vi "USRP Dummy DMA Fetch Whatever (Host).vi"() -> ()   [LabVIEW 2016]
uses:
  <vilib>/userdefined/High Color/nirio_resource_hc.ctl
  <vilib>/FPGAPlugInAG/USRP 294xR; 295xR 200 MSps/niLvFpga_Open_USRP 294xR; 295xR 200 MSps.vi
  <vilib>/rvi/interface/common/dynamic/niFpgaDynamicAddResources.vi
  <vilib>/FPGAPlugInAG/Dynamic/niLvFpga_Download_Dynamic.vi
  <vilib>/FPGAPlugInAG/Dynamic/niLvFpga_Run_Dynamic.vi
  <vilib>/Utility/error.llb/Error Cluster From Error Code.vi
  <vilib>/rvi/errors/niLvFpgaAdjustHostInterfaceError.vi
  <vilib>/rvi/interface/common/niFpgaWaitOnOcc.vi
  <vilib>/FPGAPlugInAG/Dynamic/niLvFpga_Close_Dynamic.vi
  <vilib>/rvi/interface/nirviOpenFPGA/nirviOpenFPGA.xnode
  FPGA Bitfiles/USRP-RIO-Streami_DummyDMA_USRPDummyv2(FPGA_kYza4iCu9yA.lvbitx
  <vilib>/rvi/interface/nirviMethod/nirviMethod.xnode
  <vilib>/rvi/interface/nirviReadWriteControl/nirviReadWriteControl.xnode
  <vilib>/rvi/interface/nirviCloseFPGA/nirviCloseFPGA.xnode
  <vilib>/rvi/errors/niLvFpgaMergeErrorWithErrorCode.vi
  <vilib>/rvi/interface/Simulation/niFpgaSimulationCallBeginRW.vi
  <instrlib>/niUsrpRio/Config/v1/Host/niUsrpRio Config v1 Host.lvlib
  NiFpgaLv.dll
  <vilib>/FPGAPlugInAG/Dynamic/niLvFpga_StopFifo_Dynamic.vi
  <vilib>/FPGAPlugInAG/Dynamic/niLvFpga_ConfigureFifo_Dynamic.vi
  <vilib>/FPGAPlugInAG/Dynamic/niLvFpga_StartFifo_Dynamic.vi
  <vilib>/FPGAPlugInAG/Dynamic/niLvFpga_ReadFifo_Dynamic.vi
panel:
  out "Host Transfer Slider":u64(slide) scale=0.0..68719476736.0
  in  "Flush FIFO?":bool
  out "Control Loop":i32
  in  "Host FIFO Max Fetch":u32=131072
  in  "Reset Host Count?":bool
  in  "Stop Transfer?":bool
  in  "Reset FPGA Count?":bool
  out "FPGA Side FIFO":cluster{u32, u32}(slide)={66, 63} scale=0.0..2047.0
  out "Host Side FIFO":cluster{u32, u32}(slide) scale=0.0..67108863.0
  out "Data Loop":i32
  out "Fetch Loop":i32
  out "Host Count":u64
  in  "Number of Samples":u64=68719476736
  out "FPGA Count":u64
  in  "Start Transfer":bool
  in  "stop":bool
  out "Elements Remaining":u32
  out "Data":u64[](array[numeric]) format="%016x"
  out "Timeout Counts":u64
  in  "Reset Timeouts?":bool
  out "Actual Depth":u32
  in  "Host Requested Depth":u32=67108864
  out "error out":errorcluster
  in  "error in (no error)":errorcluster
  in  "resource name":T1="PXI2Slot18Port1Dev1"
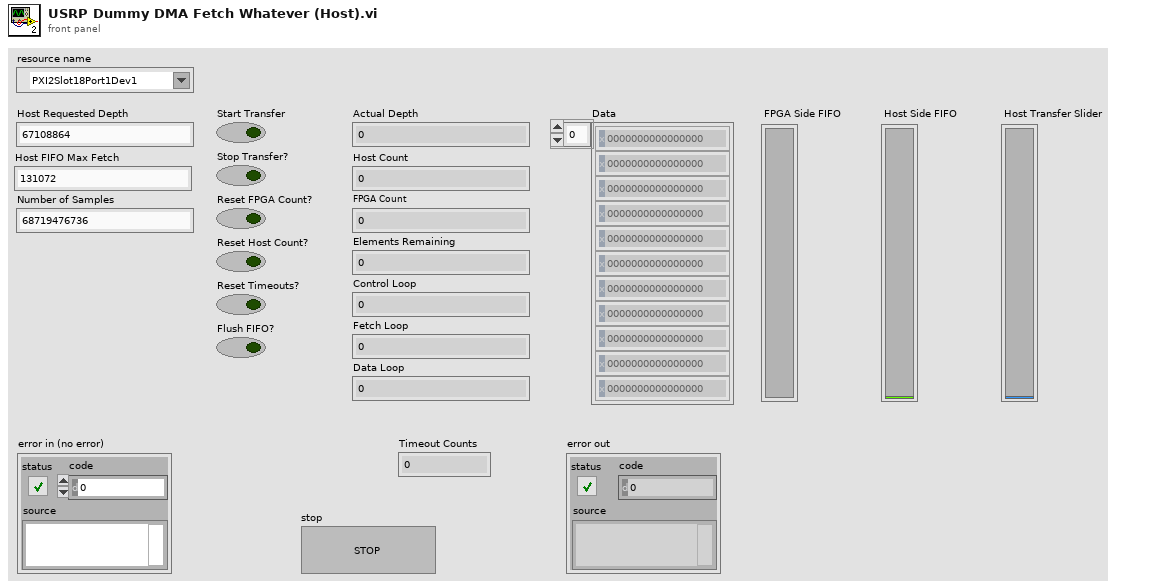
[diagram p1: front panel]
types:
  T1 = typedef "nirio_resource_hc.ctl" = tag
  T2 = typedef "niUsrpRio Config v1 Host.lvlib/niUsrpRio Session.ctl" = cluster{"FPGA Interface":refnum<k20>, "RIO Interface Number":u32, "Data Clock Rate":u32, "FPGA Data Clock Rate":u32, "Global Settings Register Bus":T3, "Radio 0 Settings Register Bus":T3, "Radio 1 Settings Register Bus":T3, "Radio Settings Bus Semaphore":T4, "DB Queues":T5[], "Characterization Data Valid?":bool, "EEPROM Header":T6, "Device Data Header":T7, "EEPROM Characterization Header":T8, "Characterization Data":T9[], "FPGA Current Version":u32, "FPGA Oldest Compatible Version":u32, "Fixed Logic Current Version":u32, "Fixed Logic Oldest Compatible Version":u32, "FPGA Radio Settings Bus Current Version":u32, "FPGA Radio Settings Bus Oldest Compatible Version":u32, "FPGA Board Config Current Version":u32, "FPGA Board Config Oldest Compatible Version":u32, "Daughterboard Clock Rate":u32, "daughterboard configuration session handles":u64[]}
  T3 = typedef "niInstr Register Bus v0 Host.lvlib/Register Bus Session.ctl" = refnum<queue>
  T4 = typedef "Semaphore RefNum" = refnum<k1>
  T5 = typedef "niUsrpRio Config v1 Host.lvlib/DB Queue Reference.ctl" = refnum<queue>
  T6 = typedef "niUsrpRio Config v1 Host.lvlib/EEPROM Header.ctl" = cluster{"Checksum":u32, "Product Code":u16, "Hardware Current Version":u16, "Hardware Oldest Compatible Version":u16, "EEPROM Map Current Version":u16, "EEPROM Map Oldest Compatible Version":u16, "User Password":string, "Pointer to Factory Header":u32, "Pointer to User Header":u32, "Recommended Interval":u16, "Number of Reserved Bytes":i32, "Number of Daughterboards":u8, "Daughterboard IDs":u16[], "Daughterboard Serial Numbers":string[]}
  T7 = typedef "niUsrpRio Config v1 Host.lvlib/EEPROM Device Data Header.ctl" = cluster{"Checksum":u32, "Number of Channels":u8, "Number of Gain Settings":u16[], "Pointer to Characterization Data":u32[], "Number of Reserved Bytes":i32, "Number of Frequencies":u16[]}
  T8 = typedef "niUsrpRio Config v1 Host.lvlib/EEPROM Characterization Header.ctl" = cluster{"Checksum":u32, "Date":timestamp, "Temperature":sgl, "Misc. Info":string, "Pointer to Device Data Header":u32, "Number of Reserved Bytes":i32}
  T9 = typedef "niUsrpRio Config v1 Host.lvlib/Characterization Data.ctl" = cluster{"Gains[dB]":dbl[], "Frequencies [Hz]":dbl[], "IQ Imbalance Table":T10[], "Measured Gains[dB]":dbl[][]}
  T10 = typedef "niUsrpRio Config v1 Host.lvlib/IQ Imbalance.ctl" = cluster{"Gain Imbalance [linear]":dbl, "Phase Imbalance [radians]":dbl, "Offset":cdb}
  T11 = cluster{"Maximum Amount Used":u32, "Current Amount Used":u32}
  T12 = cluster{"Running Max":u32, "Elements Remaining":u32}
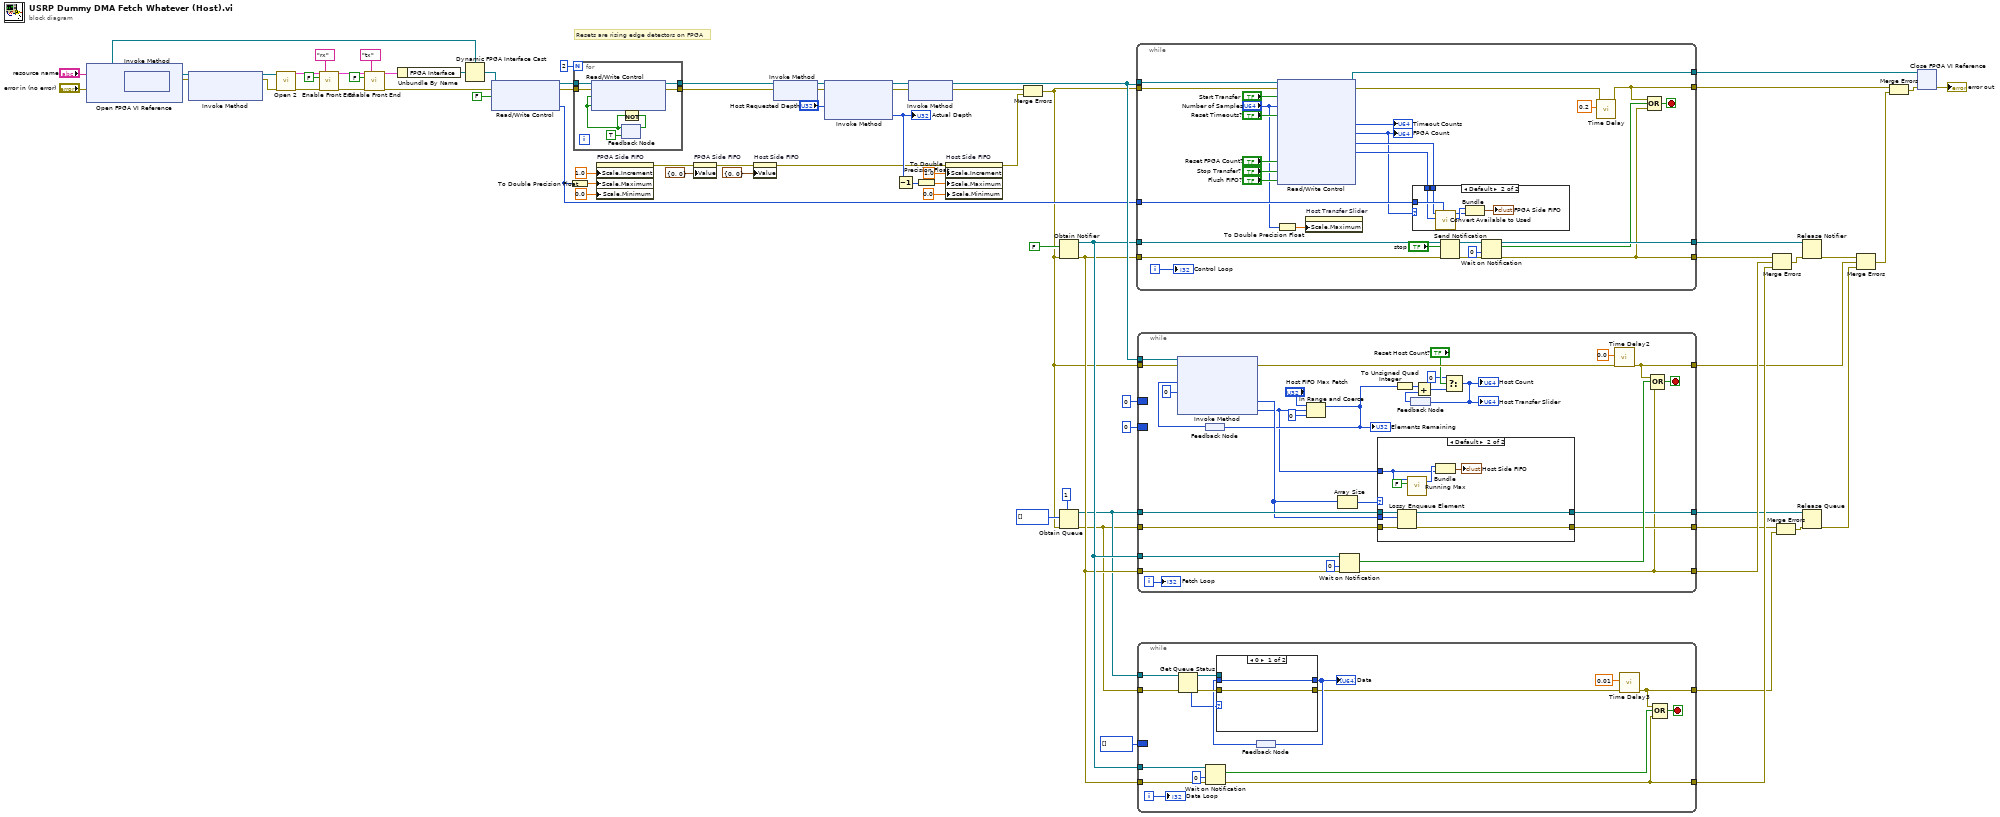
[diagram p0: block diagram]
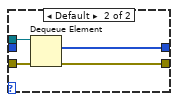
[diagram p2: hidden frame]
diagram:
  # "Resets are rising edge detectors on FPGA"
  n1 = xnode "Open FPGA VI Reference"("error in"="error in (no error)", "resource name"="resource name") -> ("FPGA VI Reference Out"=w6:refnum<k20>, "error out"=w5:errorcluster)
  n2 = xnode "Invoke Method"("FPGA VI Reference In"=w6, "error in"=w5) -> ("FPGA VI Reference Out"=w4:refnum<k20>, "error out"=w3:errorcluster)
  n3 = xnode "Invoke Method"("FPGA VI Reference In"=w4, "error in"=w3) -> ("FPGA VI Reference Out"=w2:refnum<k20>, "error out"=w1:errorcluster)  [unwired: 1 in]
  n4 = call <instrlib>:"Open 2.vi"("fpga ref"=w2, "error in"=w1) -> ("niUsrpRio Session (out)"=w65:T2, "error out"=w70:errorcluster)  [unwired: 12 in]
  n5 = call <instrlib>:"Enable Front End.vi"("niUsrpRio Session"=w65, "scope"="rx", "enable"=FALSE, "error in"=w70) -> ("niUsrpRio Session (out)"=w66:T2, "error out"=w69:errorcluster)  [unwired: 10 in]
  n6 = call <instrlib>:"Enable Front End.vi"("niUsrpRio Session"=w66, "scope"="tx", "enable"=FALSE, "error in"=w69) -> ("niUsrpRio Session (out)"=w62:T2, "error out"=w61:errorcluster)  [unwired: 10 in]
  n7 = Unbundle By Name(w62) -> ("FPGA Interface"=w60:refnum<k20>)
  n8 = Dynamic FPGA Interface Cast(Session In=w6, Type=w60) -> (Session Out=w59:refnum<k20>)
  n9 = xnode "Read/Write Control"("FPGA VI Reference In"=w59, "error in"=w61, "Start Transfer?"=FALSE ("send data?")) -> ("FPGA VI Reference Out"=w35:refnum<k20>, "error out"=w34:errorcluster, "FPGA FIFO Depth"=w20:u32)
  n10 = To Double Precision Float(number=w20) -> (double precision float=w22:dbl)
  n11 = for {
    N: 2 -> [_]
    tunnel: w35 -> [w83]
    tunnel: w34 -> [w82]
    tunnel: [w81] -> w33
    tunnel: [w80] -> w32
    n12 = feedback #1(TRUE) -> (w78:bool)
    n13 = xnode "Read/Write Control"("FPGA VI Reference In"=w83, "error in"=w82, "Reset Timeouts?"=w78, "Reset FPGA Count?"=w78) -> ("FPGA VI Reference Out"=w81:refnum<k20>, "error out"=w80:errorcluster)
    n14 = Not(x=w78) -> (.not. x?=w77:bool)
    n15 = feedback-in #1(w77) -> ()
  }
  n16 = property on="FPGA Side FIFO" class="Slide (strict)"("Scale.Increment"=1.0 ("Scale.Range:Increment"), "Scale.Maximum"=w22, "Scale.Minimum"=0.0 ("Scale.Range:Minimum")) -> (error out=w15:errorcluster)  [unwired: 2 in, 1 out]
  n17 = property on="FPGA Side FIFO" class="Slide (strict)"(error in=w15, "Value"=cluster{u32, u32} {0, 0} ("FPGA Side FIFO")) -> (error out=w18:errorcluster)  [unwired: 1 in, 1 out]
  n18 = property on="Host Side FIFO" class="Slide (strict)"(error in=w18, "Value"=cluster{u32, u32} {0, 0} ("FPGA Side FIFO")) -> (error out=w14:errorcluster)  [unwired: 1 in, 1 out]
  n19 = xnode "Invoke Method"("FPGA VI Reference In"=w33, "error in"=w32) -> ("FPGA VI Reference Out"=w76:refnum<k20>, "error out"=w75:errorcluster)
  n20 = xnode "Invoke Method"("FPGA VI Reference In"=w76, "error in"=w75, "Requested Depth"="Host Requested Depth") -> ("FPGA VI Reference Out"=w72:refnum<k20>, "error out"=w73:errorcluster, "Actual Depth"=w19:u32)
  "Actual Depth" <- w19
  n21 = Decrement(x=w19) -> (x-1=w25:u32)
  n22 = xnode "Invoke Method"("FPGA VI Reference In"=w72, "error in"=w73) -> ("FPGA VI Reference Out"=w56:refnum<k20>, "error out"=w21:errorcluster)
  n23 = To Double Precision Float(number=w25) -> (double precision float=w7:dbl)
  n24 = property on="Host Side FIFO" class="Slide (strict)"(error in=w14, "Scale.Increment"=1.0 ("Data Entry Limits:Increment"), "Scale.Maximum"=w7, "Scale.Minimum"=0.0 ("Data Entry Limits:Minimum")) -> (error out=w12:errorcluster)  [unwired: 1 in, 1 out]
  n25 = Merge Errors(w21, w12) -> (w13:errorcluster)
  n26 = Obtain Notifier(notification data type=FALSE, error in (no error)=w13) -> (notifier out=w47:refnum<notifier>, error out=w46:errorcluster)  [unwired: 2 in, 1 out]
  n27 = Obtain Queue(max queue size (-1, unlimited)=1, element data type=u64[] [] ("Data"), error in (no error)=w13) -> (queue out=w39:refnum<queue>, error out=w38:errorcluster)  [unwired: 2 in, 1 out]
  n28 = while {
    tunnel: w56 -> [w112]
    tunnel: w13 -> [w111]
    tunnel: w47 -> [w108]
    tunnel: w46 -> [w107]
    tunnel: [w102] -> w52
    tunnel: [w95] -> w51
    tunnel: [w97] -> w30
    tunnel: [w96] -> w29
    tunnel: w20 -> [w94]
    i -> [w87]
    stop <- w101 stop-if-true
    n29 = xnode "Read/Write Control"("FPGA VI Reference In"=w112, "error in"=w111, "Start Transfer?"="Start Transfer", "Number of Samples"="Number of Samples", "Reset Timeouts?"="Reset Timeouts?", "Reset FPGA Count?"="Reset FPGA Count?", "Stop Transfer?"="Stop Transfer?", "Flush FIFO?"="Flush FIFO?") -> ("FPGA VI Reference Out"=w96:refnum<k20>, "error out"=w110:errorcluster, "Timeout Count"=→"Timeout Counts":u64, "FPGA Count"=w88:u64, "Space Available"=w93:u32, "Min Space Available"=w91:u32)
    "FPGA Count" <- w88
    n30 = To Double Precision Float(number="Number of Samples") -> (double precision float=w84:dbl)
    n31 = property on="Host Transfer Slider" class="Slide (strict)"("Scale.Maximum"=w84) -> ()  [unwired: 2 in, 2 out]
    n32 = case shown="Default" w88 {
      tunnel: w94 -> [_ w118]
      tunnel: w93 -> [_ w117]
      tunnel: w91 -> [_ w116]
      frame 0 {
      }
      frame Default {
        n33 = call "Convert Available to Used.vi"("Size"=w118, "Minimum Amount Available"=w116, "Current Amount Available"=w117) -> ("Maximum Amount Used"=w115:u32, "Current Amount Used"=w114:u32)  [unwired: 5 in]
        n34 = Bundle("Maximum Amount Used"=w115, "Current Amount Used"=w114) -> (→"FPGA Side FIFO":T11)  [unwired: 1 in]
      }
    }
    n35 = Send Notification(notification="stop", notifier=w108, error in (no error)=w107) -> (notifier out=w104:refnum<notifier>, error out=w103:errorcluster)
    n36 = Wait on Notification(notifier=w104, timeout in ms (-1)=0, error in (no error)=w103) -> (notifier out=w102:refnum<notifier>, notification=w100:bool, error out=w95:errorcluster)  [unwired: 1 in, 1 out]
    n37 = call "Time Delay"("error in (no error)"=w110, "Delay Time (s)"=0.2) -> ("error out"=w97:errorcluster)  [unwired: 9 in]
    n38 = Compound Arithmetic op=OR(w97, w100, w95) -> (w101:bool)
    "Control Loop" <- w87
  }
  n39 = while {
    tunnel: [w143] -> w31
    tunnel: w56 -> [w146]
    tunnel: w13 -> [w145]
    border: u64 0 -> [_]
    border: u32 0 ("Elements Remaining") -> [_]
    tunnel: w47 -> [w139]
    tunnel: w46 -> [w138]
    tunnel: [w128] -> w49
    tunnel: [w134] -> w43
    tunnel: w39 -> [w135]
    tunnel: w38 -> [w133]
    tunnel: [w132] -> w42
    i -> [w136]
    stop <- w141 stop-if-true
    n40 = feedback #2() -> (w124:u32)
    n41 = xnode "Invoke Method"("FPGA VI Reference In"=w146, "error in"=w145, "Number of Elements"=w124, "Timeout (ms)"=0) -> ("error out"=w131:errorcluster, "Data"=w129:u64[], "Elements Remaining"=w119:u32)  [unwired: 1 out]
    n42 = In Range and Coerce(upper limit="Host FIFO Max Fetch", x=w119, lower limit=u32 0) -> (coerced(x)=w121:u32)  [unwired: 1 out]
    "Elements Remaining" <- w121
    n43 = feedback-in #2(w121) -> ()
    n44 = Array Size(array=w129) -> (size(s)=w130:i32)
    n45 = Wait on Notification(notifier=w139, timeout in ms (-1)=0, error in (no error)=w138) -> (notification=w137:bool, error out=w128:errorcluster)  [unwired: 1 in, 2 out]
    n46 = case shown="Default" w130 {
      tunnel: w135 -> [w150 w159]
      tunnel: [w150 w158] -> w134
      tunnel: w133 -> [w149 w157]
      tunnel: [w149 w156] -> w132
      tunnel: w129 -> [_ w155]
      tunnel: w119 -> [_ w151]
      frame 0 {
      }
      frame Default {
        n47 = Lossy Enqueue Element(queue=w159, element=w155, error in (no error)=w157) -> (queue out=w158:refnum<queue>, error out=w156:errorcluster)  [unwired: 2 out]
        n48 = call "Running Max.vi"("Reset"=FALSE, "Next Value"=w151) -> ("Running Max"=w152:u32)  [unwired: 5 in]
        n49 = Bundle("Running Max"=w152, "Elements Remaining"=w151) -> (→"Host Side FIFO":T12)  [unwired: 1 in]
      }
    }
    n50 = To Unsigned Quad Integer(1:w121) -> (0:w148:u64)
    n51 = feedback #3() -> (w147:u64)
    n52 = Add(x=w148, y=w147) -> (x+y=w126:u64)
    n53 = Select(t=u64 0, s="Reset Host Count?", f=w126) -> (s? t:f=w120:u64)
    "Host Count" <- w120
    "Host Transfer Slider" <- w120
    n54 = feedback-in #3(w120) -> ()
    n55 = call "Time Delay2"("error in (no error)"=w131, "Delay Time (s)"=0.0) -> ("error out"=w143:errorcluster)  [unwired: 9 in]
    n56 = Compound Arithmetic op=OR(w143, w137, w128) -> (w141:bool)
    "Fetch Loop" <- w136
  }
  n57 = while {
    tunnel: w47 -> [w174]
    tunnel: w46 -> [w173]
    tunnel: [w160] -> w45
    tunnel: w39 -> [w171]
    tunnel: w38 -> [w170]
    tunnel: [w162] -> w37
    border: u64[] [] -> [_]
    i -> [w176]
    stop <- w164 stop-if-true
    n58 = Get Queue Status(queue=w171, error in (no error)=w170) -> (queue out=w168:refnum<queue>, error out=w169:errorcluster, # elements in queue=w165:i32)  [unwired: 1 in, 5 out]
    n59 = Wait on Notification(notifier=w174, timeout in ms (-1)=0, error in (no error)=w173) -> (notification=w172:bool, error out=w160:errorcluster)  [unwired: 1 in, 2 out]
    n60 = feedback #4() -> (w167:u64[])
    n61 = case shown="0" w165 {
      tunnel: [w178 w182] -> w163
      tunnel: [w177 w179] -> w166
      tunnel: w169 -> [w178 w181]
      tunnel: w168 -> [_ w180]
      tunnel: w167 -> [w177 _]
      frame 0 {
      }
      frame Default {
        n62 = Dequeue Element(queue=w180, error in (no error)=w181) -> (element=w179:u64[], error out=w182:errorcluster)  [unwired: 1 in, 2 out]
      }
    }
    "Data" <- w166
    n63 = feedback-in #4(w166) -> ()
    n64 = call "Time Delay3"("error in (no error)"=w163, "Delay Time (s)"=0.01) -> ("error out"=w162:errorcluster)  [unwired: 9 in]
    n65 = Compound Arithmetic op=OR(w162, w172, w160) -> (w164:bool)
    "Data Loop" <- w176
  }
  n66 = Merge Errors(w51, w49, w45) -> (w50:errorcluster)
  n67 = Merge Errors(w42, w37) -> (w41:errorcluster)
  n68 = Release Notifier(notifier=w52, error in (no error)=w50) -> (error out=w48:errorcluster)  [unwired: 1 in, 2 out]
  n69 = Release Queue(queue=w43, error in (no error)=w41) -> (error out=w40:errorcluster)  [unwired: 1 in, 2 out]
  n70 = Merge Errors(w48, w31, w40) -> (w8:errorcluster)
  n71 = Merge Errors(w30, w8) -> (w9:errorcluster)
  n72 = xnode "Close FPGA VI Reference"("FPGA VI Reference In"=w29, "error in"=w9) -> ("error out"=→"error out":errorcluster)
